vi "Timing Tester master.vi"() -> ()   [LabVIEW 2015]
uses:
  <vilib>/Platform/TimedLoop/XDataNode/timing_clust.ctl
  <vilib>/Platform/TimedLoop/XDataNode/nitl_modes.ctl
  <vilib>/Platform/TimedLoop/XDataNode/wakeup.ctl
  <vilib>/rvi/Emulation/niFpgaGetClockAttributes.vi
  <vilib>/rvi/Emulation/niFpgaSctlEmulationGetInTimedLoop.vi
  <vilib>/rvi/Emulation/niFpgaEmulationReportErrorSimple.vi
  <vilib>/rvi/eio/common/nirviEmuTemplateMethod_errors.vi
  <vilib>/rvi/Emulation/niFpgaProcessEmulError.vi
  <vilib>/rvi/Emulation/niFpgaCriticalErrorInLSC.vi
  <vilib>/eio/EIONode/EIONode.xnode
  <vilib>/Platform/TimedLoop/XDataNode/XDataNode.xnode
  <vilib>/Platform/TimedLoop/XDataNode/XDNodeRunTimeDep.lvlib
panel:
  out "do":bool
  in  "AOlower limit":i16
  in  "AOupper limit":i16
  in  "DOlower limit":i16
  in  "DOupper limit":i16
  out "User Command Idle":bool
  out "User Command Status":u8
  out "User Error 2":bool
  out "Configured? 2":bool
  out "PLL Locked":bool
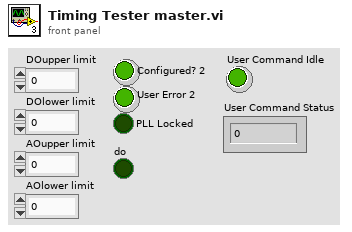
[diagram p1: front panel]
types:
  T1 = typedef "XDNodeRunTimeDep.lvlib/timing_clust.ctl" = cluster{"Expected End [f-1]":u64, "Actual End [f-1]":u64, "Finished Late? [f-1]":bool, "Expected End [i-1]":u64, "Actual End [i-1]":u64, "Finished Late? [i-1]":bool, "Expected Start [i]":u64, "Actual Start [i]":u64, "Expected Start [f]":u64, "Actual Start [f]":u64, "Source Name":string, "Structure Name":string, "Period":i64, "Deadline":i64, "Offset":i64, "Start":i64, "Priority":i32, "Timeout":i32, "Mode":T2, "Wakeup Reason":T3, "Error":errorcluster, "Source Type":string, "Secondary Source Type":string, "Global End Time":u64, "Global Start Time":u64, "Frame Duration":u64, "Iteration Duration":u64, "Assigned CPU":i32, "I/O Scan Engine Mode":u32}
  T2 = typedef "XDNodeRunTimeDep.lvlib/nitl_modes.ctl" = enum32{"No Change", "Process missed periods, maintain original phase", "Discard missed periods, maintain original phase", "Process missed periods, ignore original phase", "Discard missed periods, ignore original phase"}
  T3 = typedef "XDNodeRunTimeDep.lvlib/wakeup.ctl" = enum32{"Normal", "Aborted", "Asynchronous wakeup", "Timing source error", "Timed loop error", "Timeout"}
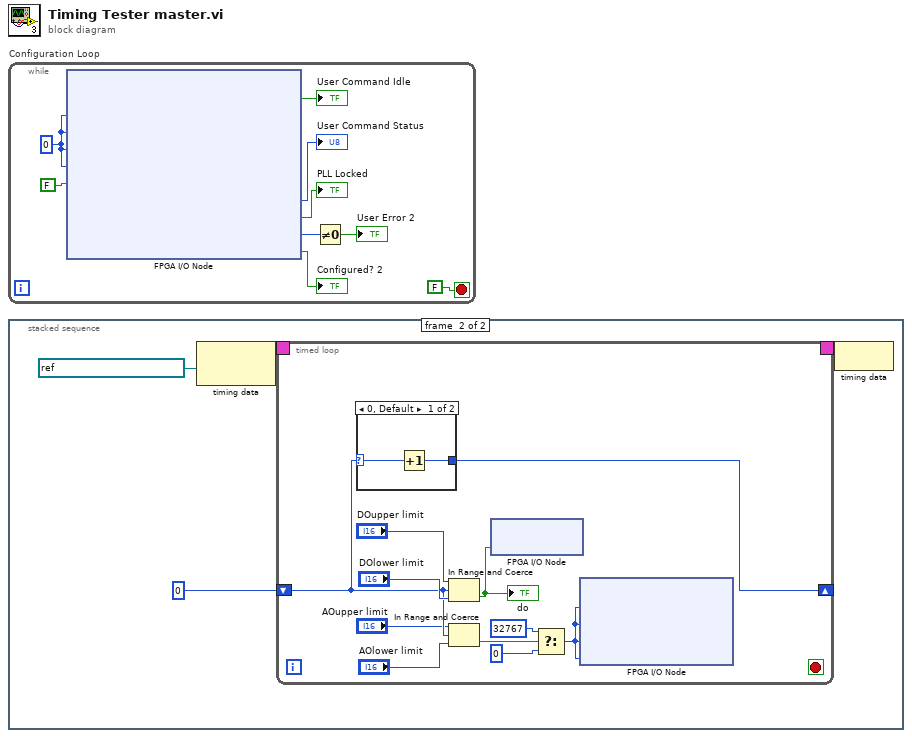
[diagram p0: block diagram]
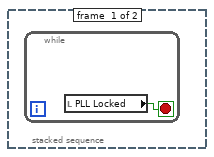
[diagram p2: hidden frame]
diagram:
  n1 = while "Configuration Loop" {
    stop <- FALSE stop-if-true
    w2 = u8 0 ("SPI Device")
    n2 = xnode "FPGA I/O Node"("IO Module\\SPI Device"=w2, "IO Module\\User Command"=w2, "IO Module\\User Data 0"=w2, "IO Module\\User Data 1"=w2, "IO Module\\User Command Commit"=FALSE ("IO Module\\User Command Commit")) -> ("IO Module\\User Command Idle"=→"User Command Idle":bool, "IO Module\\User Command Status"=→"User Command Status":u8, "IO Module\\PLL Locked"=→"PLL Locked":bool, "IO Module\\User Error"=w6:u8, "IO Module\\Initialization Done"=→"Configured? 2":bool)  [unwired: 10 in, 10 out]
    n3 = Not Equal To 0?(x=w6) -> (x != 0?=→"User Error 2":bool)
  }
  n4 = stacked-sequence {
    frame #0 {
      n5 = while {
        stop <- w10 stop-if-true
        n6 = local read "PLL Locked"() -> (w10:bool)
      }
    }
    frame #1 {
      n7 = node-c288(refnum<k21> "IO Module\\Data Clock" ("Source Name")) -> (w14:T1)
      n8 = timed-loop {
        timing: w14 -> [_]
        timing-out: [_] -> w13
        shift-right: [w25] -> _
        shift-left: i16 0 -> [w17]
        stop <- _ stop-if-true
        n9 = case shown="0, Default" w17 {
          selector: w17 -> [w27 _]
          tunnel: [w26 _] -> w25
          frame 0, Default {
            n10 = Increment(x=w27) -> (x+1=w26:i16)
          }
          frame 99 {
          }
        }
        n11 = In Range and Coerce(upper limit="DOupper limit", x=w17, lower limit="DOlower limit") -> (In Range?=w22:bool)  [unwired: 1 out]
        "do" <- w22
        n12 = In Range and Coerce(upper limit="AOupper limit", x=w17, lower limit="AOlower limit") -> (In Range?=w21:bool)  [unwired: 1 out]
        n13 = xnode "FPGA I/O Node"("PXI_Trig0"=w22) -> ()  [unwired: 1 in, 1 out]
        n14 = Select(t=i16 32767 ("IO Module\\AO 0 N"), s=w21, f=i16 0 ("IO Module\\AO 0 N")) -> (s? t:f=w18:i16)
        n15 = xnode "FPGA I/O Node"("IO Module\\AO 0 N-3"=w18, "IO Module\\AO 0 N-2"=w18, "IO Module\\AO 0 N-1"=w18, "IO Module\\AO 0 N"=w18) -> ()  [unwired: 4 in, 4 out]
      }
      n16 = node-c288(w13) -> ()
    }
  }
